vi "NI OCR-Search Ctl Label By Reference.vi"(8 "error in":errorcluster, 10 "Ctl Refnum In":refnum<vi>, 11 "Buffer Data In":T1={"VI Refnum"=refnum, "Src Image"=refnum, "Dst Image"=refnum, "Ctl Refnum []"=[], "Ctl Label"=[], "User Event"=refnum, "Event Registration Refnum"=refnum, "Timeout"=0, "IMAQ OCR Session"=refnum, "Objects"=[], "ROI Descriptor"={"Global Rectangle"=[], "Contours"=[]}, "Settings"={"Objects"=0, "Threshold"=128, "Reject Border"=FALSE, "Fill Holes"=FALSE, "Min Object Size"=FALSE, "Min Size"=3, "Max Object Size"=FALSE, "Max Size"=100, "Show Search Area"=FALSE, "Show Center"=TRUE, "Show Bounding Box"=TRUE}} {"Settings"."Objects" items=["Bright Objects", "Dark Objects"]; "Settings"."Threshold" min=1 max=999999999 step=1; "Settings"."Max Size" min=1 max=999999999 step=1; "Settings"."Min Size" min=1 max=999999999 step=1; "ROI Descriptor"."Contours"."Type" items=["No Selection", "Point", "Line", "Rectangle", "Oval", "Polygon", "Freehand Region", "Annulus", "Unused2", "Unused3", "Broken Line", "Freehand Line", "Rotated Rectangle"]; "Objects"."Aspect Ratio" format="%.2f"; "Objects"."Orientation" format="%.2f"; "Objects"."Area" format="%.2f"; "Objects"."Object Center"."Y" format="%.2f"; "Objects"."Object Center"."X" format="%.2f"}) -> (0 "error out":errorcluster, 1 "Ctl Label":string, 2 "Ctl Refnum Out":refnum<vi>, 3 "Buffer Data Out":T1={"VI Refnum"=refnum, "Src Image"=refnum, "Dst Image"=refnum, "Ctl Refnum []"=[], "Ctl Label"=[], "User Event"=refnum, "Event Registration Refnum"=refnum, "Timeout"=0, "IMAQ OCR Session"=refnum, "Objects"=[], "ROI Descriptor"={"Global Rectangle"=[], "Contours"=[]}, "Settings"={"Objects"=0, "Threshold"=128, "Reject Border"=FALSE, "Fill Holes"=FALSE, "Min Object Size"=FALSE, "Min Size"=3, "Max Object Size"=FALSE, "Max Size"=100, "Show Search Area"=FALSE, "Show Center"=TRUE, "Show Bounding Box"=TRUE}} {"Settings"."Objects" items=["Bright Objects", "Dark Objects"]; "Settings"."Threshold" min=1 max=999999999 step=1; "Settings"."Max Size" min=1 max=999999999 step=1; "Settings"."Min Size" min=1 max=999999999 step=1; "ROI Descriptor"."Contours"."Type" items=["No Selection", "Point", "Line", "Rectangle", "Oval", "Polygon", "Freehand Region", "Annulus", "Unused2", "Unused3", "Broken Line", "Freehand Line", "Rotated Rectangle"]; "Objects"."Aspect Ratio" format="%.2f"; "Objects"."Orientation" format="%.2f"; "Objects"."Area" format="%.2f"; "Objects"."Object Center"."Y" format="%.2f"; "Objects"."Object Center"."X" format="%.2f"})   [LabVIEW 2016]
uses:
  Data Def/NI OCR-Buffer Data.ctl
  <vilib>/vision/Image Controls.llb/IMAQ Image.ctl
  Data Def/NI OCR-User Event Data.ctl
  <vilib>/vision/OCR.llb/IMAQ OCR Session.ctl
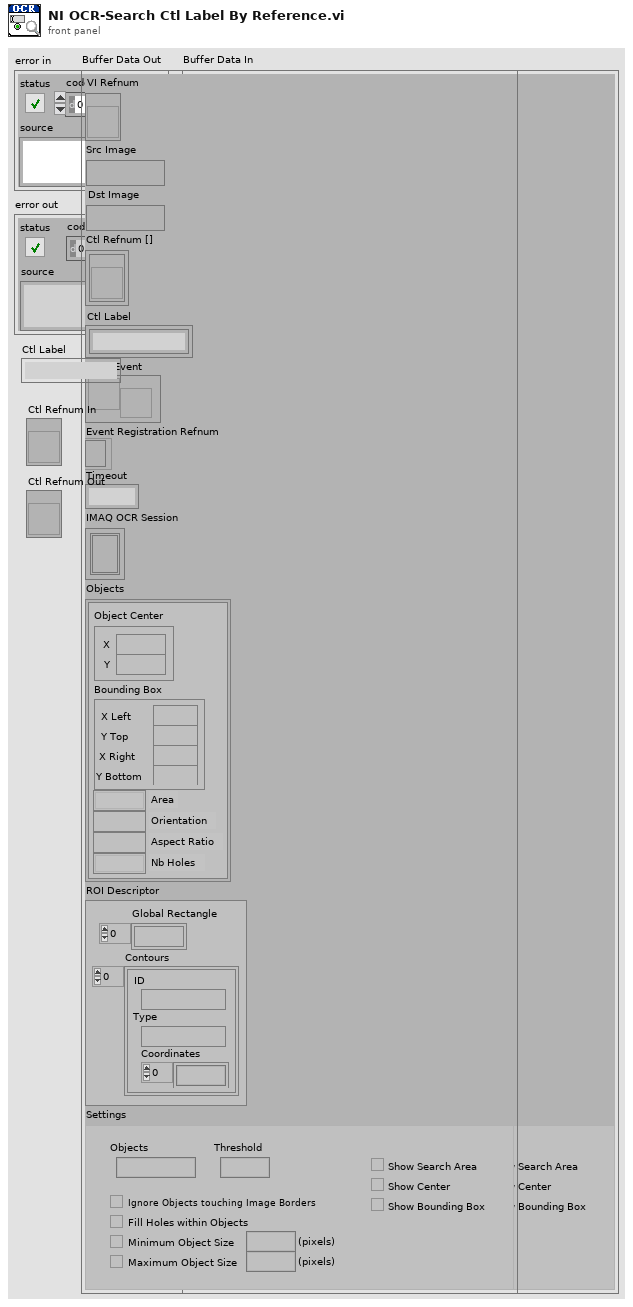
[diagram p1: front panel]
types:
  T1 = typedef "NI OCR-Buffer Data.ctl" = cluster{"VI Refnum":refnum<vi>, "Src Image":T2, "Dst Image":T2, "Ctl Refnum []":refnum<vi>[], "Ctl Label":string[], "User Event":refnum<user-event>, "Event Registration Refnum":refnum<event-registration>, "Timeout":i32, "IMAQ OCR Session":T3, "Objects":cluster{"Object Center":cluster{"X":sgl, "Y":sgl}, "Bounding Box":cluster{"X Left":i32, "Y Top":i32, "X Right":i32, "Y Bottom":i32}, "Area":sgl, "Orientation":sgl, "Aspect Ratio":sgl, "Nb Holes":i32}[], "ROI Descriptor":T4, "Settings":cluster{"Objects":u16, "Threshold":i32, "Reject Border":bool, "Fill Holes":bool, "Min Object Size":bool, "Min Size":i32, "Max Object Size":bool, "Max Size":i32, "Show Search Area":bool, "Show Center":bool, "Show Bounding Box":bool}}
  T2 = typedef "IMAQ Image.ctl" = refnum<image>
  T3 = typedef "IMAQ OCR Session.ctl" = refnum<k1>
  T4 = typedef "ROI Descriptor" = cluster{"Global Rectangle":i32[], "Contours":cluster{"ID":enum32{"External", "Internal"}, "Type":u32, "Coordinates":i32[]}[]}
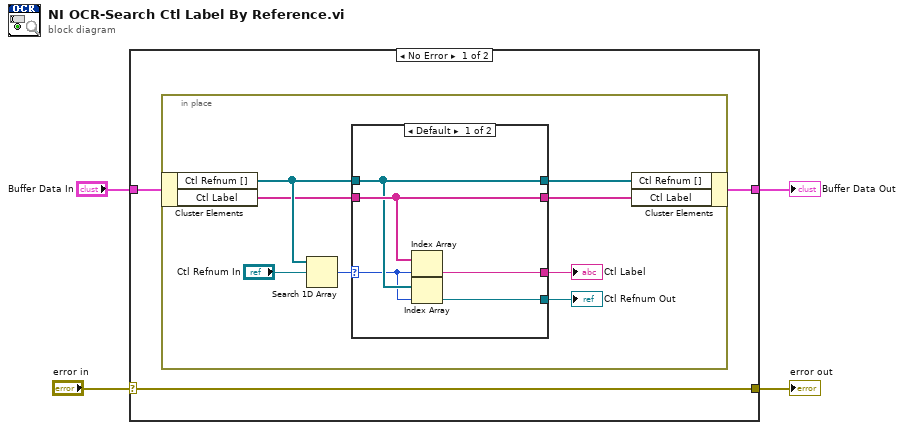
[diagram p0: block diagram]
diagram:
  n1 = case shown="No Error" "error in" {
    selector: "error in" -> [w5 w24]
    tunnel: "Buffer Data In" -> [w7 w23]
    tunnel: [w6 w23] -> w3
    tunnel: [w5 w24] -> w1
    frame No Error {
      n2 = in-place {
        n3 = in-place-cluster #1(w7) -> ("Ctl Refnum []"=w13:refnum<vi>[], "Ctl Label"=w12:string[])
        n4 = Search 1D Array(1D array=w13, element="Ctl Refnum In") -> (index of element=w10:i32)  [unwired: 1 in]
        n5 = case shown="Default" w10 {
          selector: w10 -> [w17 _]
          tunnel: [w18 w22] -> w14
          tunnel: w13 -> [w18 w22]
          tunnel: w12 -> [w20 w21]
          tunnel: [w20 w21] -> w11
          tunnel: [w19 _] -> w9
          tunnel: [w16 _] -> w8
          frame Default {
            n6 = Index Array(array=w20, index=w17) -> (element=w19:string)
            n7 = Index Array(array=w18, index=w17) -> (element=w16:refnum<vi>)
          }
          frame -1 {
          }
        }
        "Ctl Label" <- w9
        "Ctl Refnum Out" <- w8
        n8 = in-place-cluster #1("Ctl Refnum []"=w14, "Ctl Label"=w11) -> (w6:T1)
      }
    }
    frame Error {
    }
  }
  "error out" <- w1
  "Buffer Data Out" <- w3
